vi "Unescape HTTP URL.vi"(1 "escaped string in":string) -> (0 "unescaped string out":string)   [LabVIEW 2017]
uses:
  <vilib>/wsapi/NI_WebServices.lvlib
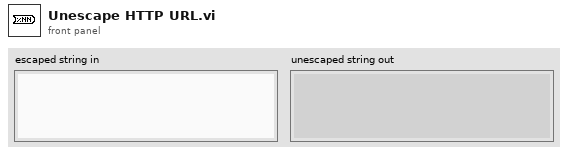
[diagram p1: front panel]
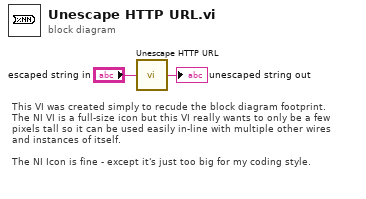
[diagram p0: block diagram]
diagram:
  # "This VI was created simply to recude the block diagram footprint.\nThe NI VI is a full-size icon but this VI really wants to only be a few\npixels tall so it can be used easily in-line with multiple other wires\nand instances of itself.\n\nThe NI Icon is fine - except it's just too big for my coding style."
  n1 = call <vilib>:"Unescape HTTP URL.vi"("escaped string in"="escaped string in") -> ("unescaped string out"=→"unescaped string out":string)
